vi "LoggigProgram.vi"() -> ()   [LabVIEW 2020]
uses:
  <vilib>/xnet/xnet.llb/XNET Create Session (Frame Output Stream).vi
  <vilib>/xnet/xnet.llb/XNET Write (Frame CAN).vi
  <vilib>/xnet/xnet.llb/XNET Create Session (Frame Input Stream).vi
  <vilib>/xnet/xnet.llb/XNET Read (Frame CAN).vi
  <resource>/objmgr/xnet.rc
panel:
  in  "stop":bool
  out "outputIMUData":T1
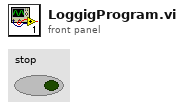
[diagram p1: front panel]
types:
  T1 = cluster{"ID1":cluster{"Accerlation-X(g)":dbl, "Accerlation-Y(g)":dbl, "Accerlation-Z(g)":dbl, "AngularPosition-X(g)":dbl, "AngularPosition-Y(g)":dbl, "AngularPosition-Z(g)":dbl}, "ID2":cluster{"Accerlation-X(g)":dbl, "Accerlation-Y(g)":dbl, "Accerlation-Z(g)":dbl, "AngularPosition-X(g)":dbl, "AngularPosition-Y(g)":dbl, "AngularPosition-Z(g)":dbl}, "ID3":cluster{"Accerlation-X(g)":dbl, "Accerlation-Y(g)":dbl, "Accerlation-Z(g)":dbl, "AngularPosition-X(g)":dbl, "AngularPosition-Y(g)":dbl, "AngularPosition-Z(g)":dbl}}
  T2 = cluster{"RelativeTime(sec)":dbl, "outputIMUData":cluster{"ID1":cluster{"Accerlation-X(g)":dbl, "Accerlation-Y(g)":dbl, "Accerlation-Z(g)":dbl, "AngularPosition-X(g)":dbl, "AngularPosition-Y(g)":dbl, "AngularPosition-Z(g)":dbl}, "ID2":cluster{"Accerlation-X(g)":dbl, "Accerlation-Y(g)":dbl, "Accerlation-Z(g)":dbl, "AngularPosition-X(g)":dbl, "AngularPosition-Y(g)":dbl, "AngularPosition-Z(g)":dbl}, "ID3":cluster{"Accerlation-X(g)":dbl, "Accerlation-Y(g)":dbl, "Accerlation-Z(g)":dbl, "AngularPosition-X(g)":dbl, "AngularPosition-Y(g)":dbl, "AngularPosition-Z(g)":dbl}}}
  T3 = enum16{"open", "replace", "create", "open or create", "replace or create", "replace or create with confirmation"}
  T4 = typedef "XNET Frame CAN.ctl" = cluster{"timestamp":timestamp, "payload":u8[], "identifier":u32, "type":T5, "extended?":bool, "echo?":bool}
  T5 = typedef "XNET Frame Type CAN.ctl" = u8
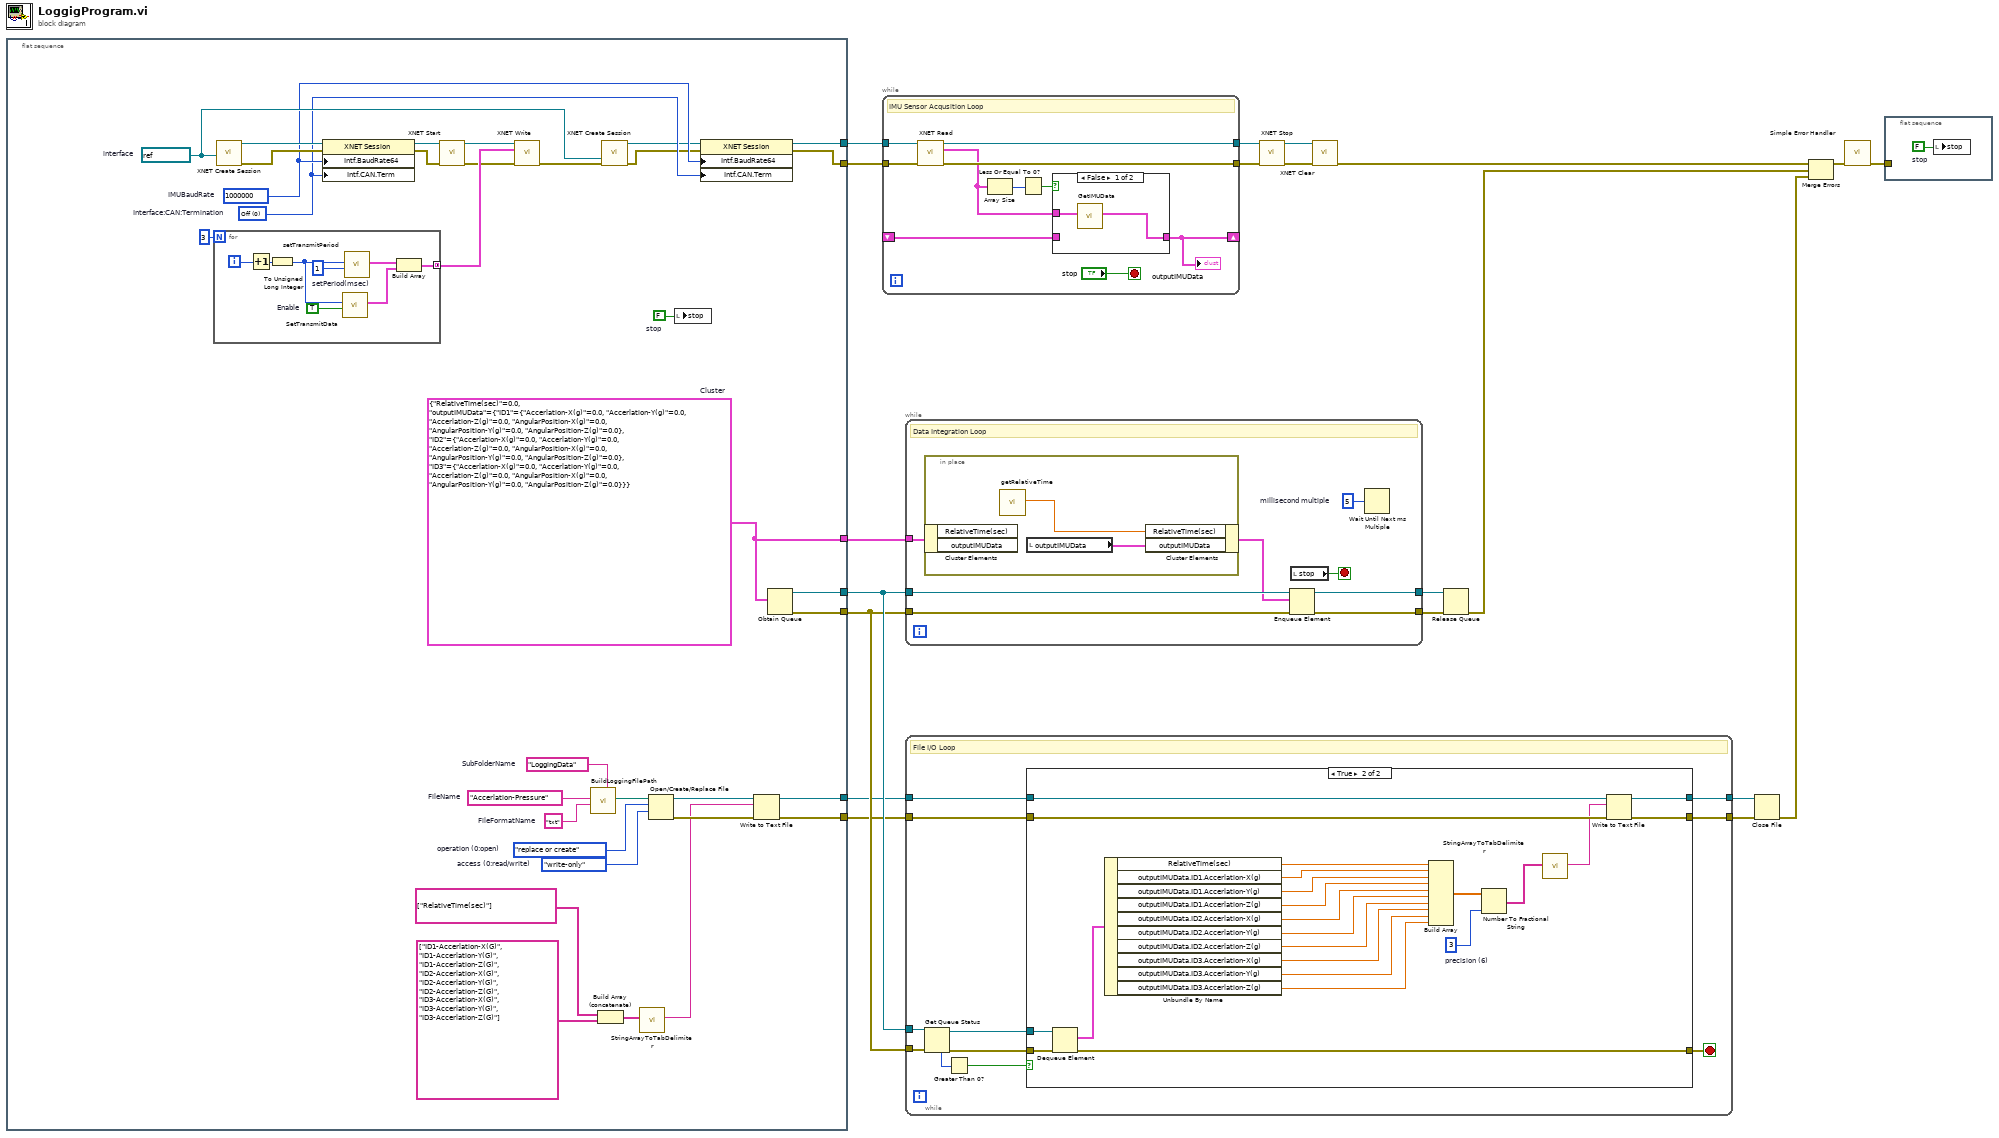
[diagram p0: block diagram]
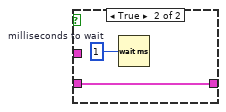
[diagram p2: hidden frame]
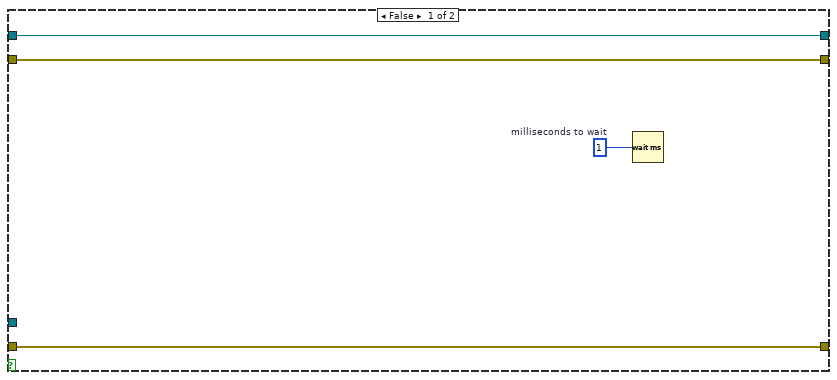
[diagram p3: hidden frame]
diagram:
  n1 = flat-sequence {
    tunnel: [w45] -> w20
    tunnel: [w44] -> w19
    tunnel: [w38] -> w12
    tunnel: [w37] -> w9
    tunnel: [w36] -> w8
    tunnel: [w28] -> w5
    tunnel: [w26] -> w4
    frame #0 {
      w49 = u64 1000000  # IMUBaudRate
      w38 = T2 {"RelativeTime(sec)"=0.0, "outputIMUData"={"ID1"={"Accerlation-X(g)"=0.0, "Accerlation-Y(g)"=0.0, "Accerlation-Z(g)"=0.0, "AngularPosition-X(g)"=0.0, "AngularPosition-Y(g)"=0.0, "AngularPosition-Z(g)"=0.0}, "ID2"={"Accerlation-X(g)"=0.0, "Accerlation-Y(g)"=0.0, "Accerlation-Z(g)"=0.0, "AngularPosition-X(g)"=0.0, "AngularPosition-Y(g)"=0.0, "AngularPosition-Z(g)"=0.0}, "ID3"={"Accerlation-X(g)"=0.0, "Accerlation-Y(g)"=0.0, "Accerlation-Z(g)"=0.0, "AngularPosition-X(g)"=0.0, "AngularPosition-Y(g)"=0.0, "AngularPosition-Z(g)"=0.0}}}  # Cluster
      w30 = enum16{"read/write", "read-only", "write-only"}."write-only"  # access (0:read/write)
      w31 = T3."replace or create"  # operation (0:open)
      w33 = "txt"  # FileFormatName
      w34 = "Accerlation-Pressure"  # FileName
      w35 = "LoggingData"  # SubFolderName
      w21 = FALSE  # stop
      w48 = u32 0 items=["Off", "On"]  # Interface:CAN:Termination
      w50 = refnum<k21> "CAN1"  # interface
      n2 = for {
        N: 3 -> [_]
        tunnel: [w59] -> w51 mode=concatenating
        i -> [w57]
        w58 = TRUE  # Enable
        w62 = u32 1  # setPeriod(msec)
        n3 = Increment(x=w57) -> (x+1=w56:i32)
        n4 = To Unsigned Long Integer(number=w56) -> (unsigned 32bit integer=w55:u32)
        n5 = call "SetTransmitData.vi"("Enable"=w58, "identifier"=w55) -> ("outputCANFrame"=w60:T4)  [unwired: 9 in]
        n6 = call "setTransmitPeriod.vi"("setPeriod(msec)"=w62, "identifier"=w55) -> ("outputCANFrame"=w61:T4)  [unwired: 9 in]
        n7 = Build Array(w61, w60) -> (w59:T4[])
      }
      n8 = call-poly <vilib>:"XNET Create Session.vi"("interface"=w50) -> ("session out"=w54:refnum<k21>, "error out"=w53:errorcluster)  [unwired: 13 in]
      n9 = property class="XNET Session"(reference=w54, error in=w53, "Intf.BaudRate64"=w49, "Intf.CAN.Term"=w48) -> (reference out=w52:refnum<k21>, error out=w42:errorcluster)
      n10 = call <vilib>:"XNET Start.vi"("session in"=w52, "error in (no error)"=w42) -> ("session out"=w43:refnum<k21>, "error out"=w41:errorcluster)  [unwired: 12 in]
      n11 = call-poly <vilib>:"XNET Write.vi"("session in"=w43, "data"=w51, "error in (no error)"=w41) -> ("error out"=w40:errorcluster)  [unwired: 11 in, 1 out]
      n12 = call "BuildLoggingFilePath.vi"("SubFolderName"=w35, "FileFormatName"=w33, "FileName"=w34) -> ("appended path"=w32:path)  [unwired: 8 in]
      n13 = Build Array (concatenate) "Build Array"(string[] ["RelativeTime(sec)"], string[] ["ID1-Accerlation-X(G)", "ID1-Accerlation-Y(G)", "ID1-Accerlation-Z(G)", "ID2-Accerlation-X(G)", "ID2-Accerlation-Y(G)", "ID2-Accerlation-Z(G)", "ID3-Accerlation-X(G)", "ID3-Accerlation-Y(G)", "ID3-Accerlation-Z(G)"]) -> (w23:string[])
      n14 = call-poly <vilib>:"XNET Create Session.vi"("interface"=w50, "error in (no error)"=w40) -> ("session out"=w47:refnum<k21>, "error out"=w46:errorcluster)  [unwired: 12 in]
      n15 = call "StringArrayToTabDelimiter.vi"("StringArray"=w23) -> ("String"=w22:string)  [unwired: 10 in]
      n16 = Open/Create/Replace File(file path (use dialog)=w32, operation (0:open)=w31, access (0:read/write)=w30) -> (refnum out=w29:refnum<file>, error out=w27:errorcluster)  [unwired: 3 in, 1 out]
      n17 = local write "stop"(w21) -> ()
      n18 = property class="XNET Session"(reference=w47, error in=w46, "Intf.BaudRate64"=w49, "Intf.CAN.Term"=w48) -> (reference out=w45:refnum<k21>, error out=w44:errorcluster)
      n19 = Write to Text File(file (use dialog)=w29, text=w22, error in=w27) -> (refnum out=w28:refnum<file>, error out=w26:errorcluster)  [unwired: 1 in, 1 out]
      n20 = Obtain Queue(element data type=w38) -> (queue out=w37:refnum<queue>, error out=w36:errorcluster)  [unwired: 4 in, 1 out]
    }
  }
  n21 = while {
    shift-right: [w65] -> _
    shift-left: _ -> [w64]
    tunnel: w20 -> [w72]
    tunnel: [w70] -> w18
    tunnel: w19 -> [w71]
    tunnel: [w69] -> w16
    stop <- "stop" stop-if-true
    # "IMU Sensor Acqusition Loop"
    n22 = call-poly <vilib>:"XNET Read.vi"("session in"=w72, "error in (no error)"=w71) -> ("session out"=w70:refnum<k21>, "data"=w68:T4[], "error out"=w69:errorcluster)  [unwired: 10 in, 1 out]
    n23 = Array Size(array=w68) -> (size(s)=w67:i32)
    n24 = Less Or Equal To 0?(x=w67) -> (x <= 0?=w66:bool)
    n25 = case shown="False" w66 {
      tunnel: w68 -> [w74 _]
      tunnel: [w73 w75] -> w65
      tunnel: w64 -> [_ w75]
      frame False {
        n26 = call "GetIMUData.vi"("InputCANData"=w74) -> ("outputIMUData"=w73:T1)  [unwired: 10 in]
      }
      frame True {
        w76 = u32 1  # milliseconds to wait
        n27 = Wait (ms)(milliseconds to wait=w76) -> ()  [unwired: 1 out]
      }
    }
    "outputIMUData" <- w65
  }
  n28 = while {
    tunnel: w9 -> [w83]
    tunnel: w12 -> [w82]
    tunnel: w8 -> [w80]
    tunnel: [w79] -> w11
    tunnel: [w78] -> w10
    stop <- w84 stop-if-true
    w77 = u32 5  # millisecond multiple
    # "Data Integration Loop"
    n29 = in-place {
      n30 = in-place-cluster #1(w82) -> ()  [unwired: 2 out]
      n31 = call "getRelativeTime.vi"() -> ("getRelativeTime(sec)"=w85:dbl)  [unwired: 11 in]
      n32 = local read "outputIMUData"() -> (w86:T1)
      n33 = in-place-cluster #1("RelativeTime(sec)"=w85, "outputIMUData"=w86) -> (w81:T2)
    }
    n34 = Enqueue Element(queue=w83, element=w81, error in (no error)=w80) -> (queue out=w79:refnum<queue>, error out=w78:errorcluster)  [unwired: 1 in, 1 out]
    n35 = local read "stop"() -> (w84:bool)
    n36 = Wait Until Next ms Multiple(millisecond multiple=w77) -> ()  [unwired: 1 out]
  }
  n37 = while {
    tunnel: w9 -> [w97]
    tunnel: w8 -> [w96]
    tunnel: w5 -> [w90]
    tunnel: w4 -> [w89]
    tunnel: [w88] -> w3
    tunnel: [w87] -> w2
    stop <- w91 stop-if-true
    # "File I/O Loop"
    n38 = Get Queue Status(queue=w97, error in (no error)=w96) -> (queue out=w93:refnum<queue>, error out=w92:errorcluster, # elements in queue=w95:i32)  [unwired: 1 in, 5 out]
    n39 = Greater Than 0?(x=w95) -> (x > 0?=w94:bool)
    n40 = case shown="True" w94 {
      tunnel: w93 -> [_ w123]
      tunnel: w92 -> [w101 w122]
      tunnel: [w101 w121] -> w91
      tunnel: w90 -> [w100 w120]
      tunnel: w89 -> [w99 w119]
      tunnel: [w100 w118] -> w88
      tunnel: [w99 w117] -> w87
      frame False {
        w98 = u32 1  # milliseconds to wait
        n41 = Wait (ms)(milliseconds to wait=w98) -> ()  [unwired: 1 out]
      }
      frame True {
        w105 = i16 3  # precision (6)
        n42 = Dequeue Element(queue=w123, error in (no error)=w122) -> (element=w116:T2, error out=w121:errorcluster)  [unwired: 1 in, 2 out]
        n43 = Unbundle By Name(w116) -> ("RelativeTime(sec)"=w103:dbl, "outputIMUData.ID1.Accerlation-X(g)"=w115:dbl, "outputIMUData.ID1.Accerlation-Y(g)"=w114:dbl, "outputIMUData.ID1.Accerlation-Z(g)"=w113:dbl, "outputIMUData.ID2.Accerlation-X(g)"=w112:dbl, "outputIMUData.ID2.Accerlation-Y(g)"=w111:dbl, "outputIMUData.ID2.Accerlation-Z(g)"=w110:dbl, "outputIMUData.ID3.Accerlation-X(g)"=w109:dbl, "outputIMUData.ID3.Accerlation-Y(g)"=w108:dbl, "outputIMUData.ID3.Accerlation-Z(g)"=w107:dbl)
        n44 = Build Array "Build Array"(w103, w115, w114, w113, w112, w111, w110, w109, w108, w107) -> (w106:dbl[])
        n45 = Number To Fractional String(number=w106, precision (6)=w105) -> (F-format string=w102:string[])  [unwired: 2 in]
        n46 = call "StringArrayToTabDelimiter.vi"("StringArray"=w102) -> ("String"=w104:string)  [unwired: 10 in]
        n47 = Write to Text File(file (use dialog)=w120, text=w104, error in=w119) -> (refnum out=w118:refnum<file>, error out=w117:errorcluster)  [unwired: 1 in, 1 out]
      }
    }
  }
  n48 = call <vilib>:"XNET Stop.vi"("session in"=w18, "error in (no error)"=w16) -> ("session out"=w14:refnum<k21>, "error out"=w15:errorcluster)  [unwired: 12 in]
  n49 = call <vilib>:"XNET Clear.vi"("session in"=w14, "error in (no error)"=w15) -> ("error out"=w17:errorcluster)  [unwired: 13 in]
  n50 = Release Queue(queue=w11, error in (no error)=w10) -> (error out=w6:errorcluster)  [unwired: 1 in, 2 out]
  n51 = Close File(refnum=w3, error in=w2) -> (error out=w1:errorcluster)  [unwired: 1 out]
  n52 = Merge Errors "Merge Errors"(w17, w6, w1) -> (w7:errorcluster)
  n53 = call <vilib>:"Simple Error Handler.vi"("error in (no error)"=w7) -> ("error out"=w13:errorcluster)  [unwired: 4 in, 4 out]
  n54 = flat-sequence {
    tunnel: w13 -> [_]
    frame #0 {
      w124 = FALSE  # stop
      n55 = local write "stop"(w124) -> ()
    }
  }
